vi "Open Audio File Read (UTF-8).vi"(8 "error in (no error)":errorcluster, 11 "Path":string) -> (0 "error out":errorcluster, 3 "Audio File Refnum":T1)   [LabVIEW 2020, in "G-Audio.lvlib"]
doc: "Opens an audio file and initializes the relevant decoder.\n\nSupported codecs: flac, mp3, vorbis (ogg), and wav."
uses:
  G-Audio.lvlib
  Controls/Audio File Refnum.ctl
  Private/Result To Error.vi
  Private/Value To Audio File Refnum.vi
  <vilib>/Utility/error.llb/Error Cluster From Error Code.vi
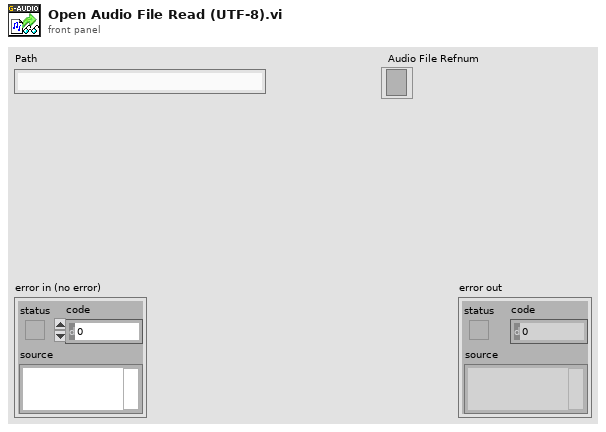
[diagram p1: front panel]
types:
  T1 = typedef "G-Audio.lvlib/Audio File Refnum.ctl" = refnum<file>
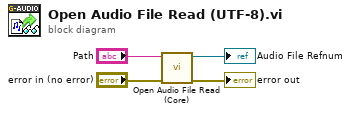
[diagram p0: block diagram]
diagram:
  n1 = call "Open Audio File Read (Core).vi"("error in (no error)"="error in (no error)", "Path"="Path") -> ("error out"=→"error out":errorcluster, "Audio File Refnum"=→"Audio File Refnum":T1)  [unwired: 8 in]
